vi "Set Shooter 2 RPM.vi"(8 "Open Loop":bool, 9 "Increment":bool, 10 "Decrement":bool, 11 "Shooter Enabled":bool) -> ()   [LabVIEW 2012]
uses:
  System Set Points and States.vi
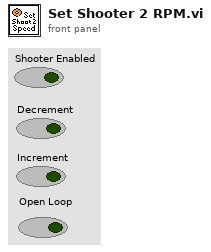
[diagram p1: front panel]
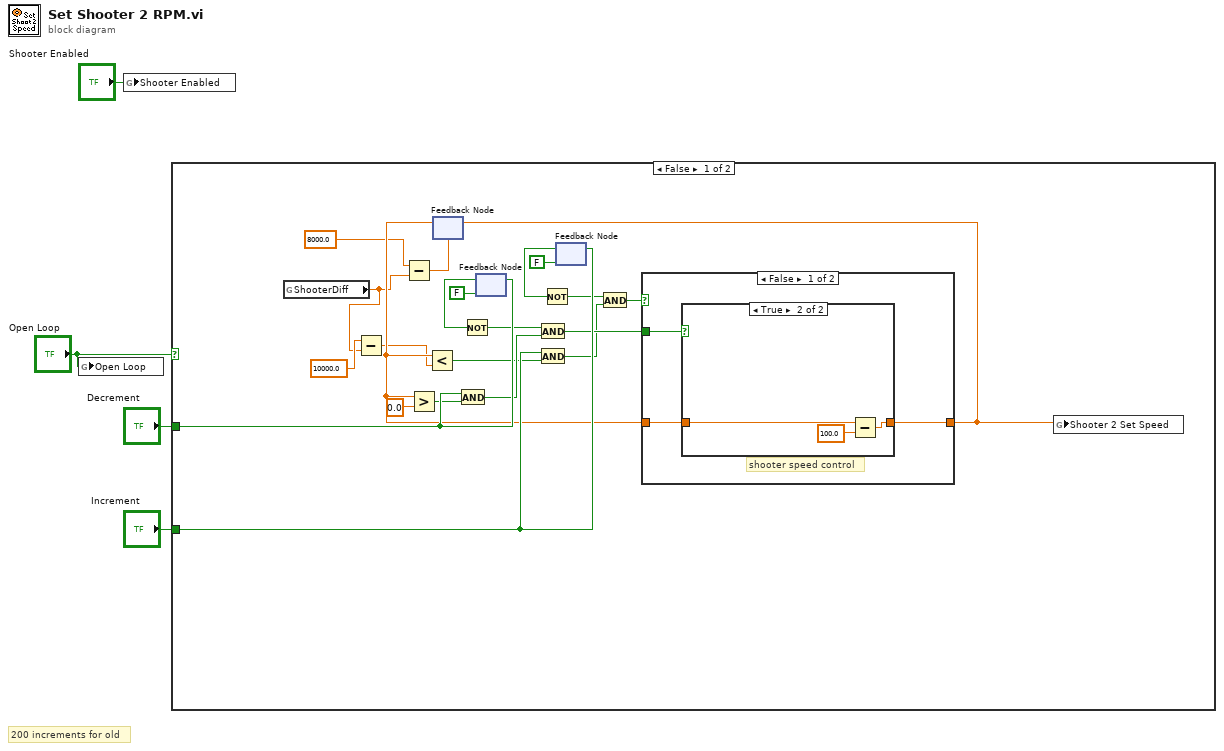
[diagram p0: block diagram]
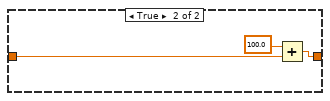
[diagram p3: hidden frame]
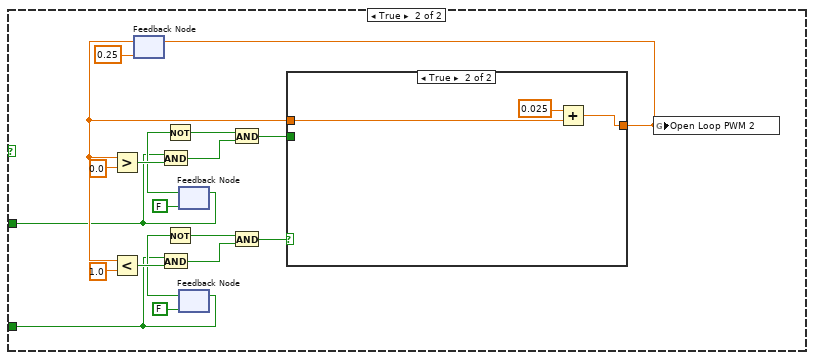
[diagram p4: hidden frame]
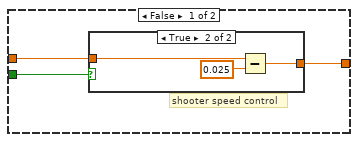
[diagram p5: hidden frame]
diagram:
  # "200 increments for old"
  n1 = global write "System Set Points and States.vi" "Open Loop"("Open Loop") -> ()
  n2 = global write "System Set Points and States.vi" "Shooter Enabled"("Shooter Enabled") -> ()
  n3 = case shown="False" "Open Loop" {
    tunnel: "Decrement" -> [w26 w39]
    tunnel: "Increment" -> [w25 w38]
    frame False {
      n4 = global read "System Set Points and States.vi" "ShooterDiff"() -> (w7:dbl)
      n5 = Subtract(x=10000.0 ("y"), y=w7) -> (x-y=w5:dbl)
      n6 = Subtract(x=8000.0, y=w7) -> (x-y=w6:dbl)
      n7 = feedback #1(w6) -> (w12:dbl)
      n8 = Greater?(x=w12, y=0.0) -> (0:w10:bool)
      n9 = Less?(x=w12, y=w5) -> (x < y?=w13:bool)
      n10 = And(x=w26, y=w10) -> (x .and. y?=w17:bool)
      n11 = feedback #2(FALSE) -> (w21:bool)
      n12 = Not(x=w21) -> (.not. x?=w22:bool)
      n13 = feedback-in #2(w26) -> ()
      n14 = And(x=w22, y=w17) -> (x .and. y?=w18:bool)
      n15 = And(x=w25, y=w13) -> (x .and. y?=w14:bool)
      n16 = feedback #3(FALSE) -> (w19:bool)
      n17 = Not(x=w19) -> (.not. x?=w20:bool)
      n18 = feedback-in #3(w25) -> ()
      n19 = And(x=w20, y=w14) -> (x .and. y?=w15:bool)
      n20 = case shown="False" w15 {
        tunnel: w18 -> [w29 _]
        tunnel: w12 -> [w28 w36]
        tunnel: [w27 w34] -> w24
        frame False {
          # "shooter speed control"
          n21 = case shown="True" w29 {
            tunnel: w28 -> [w30 w33]
            tunnel: [w30 w31] -> w27
            frame False {
            }
            frame True {
              n22 = Subtract(x=w33, y=100.0) -> (x-y=w31:dbl)
            }
          }
        }
        frame True {
          n23 = Add(x=100.0, y=w36) -> (x+y=w34:dbl)
        }
      }
      n24 = feedback-in #1(w24) -> ()
      n25 = global write "System Set Points and States.vi" "Shooter 2 Set Speed"(w24) -> ()
    }
    frame True {
      n26 = feedback #4(0.25) -> (w42:dbl)
      n27 = Greater?(x=w42, y=0.0) -> (0:w55:bool)
      n28 = Less?(x=w42, y=1.0) -> (x < y?=w53:bool)
      n29 = And(x=w39, y=w55) -> (x .and. y?=w48:bool)
      n30 = And(x=w38, y=w53) -> (x .and. y?=w50:bool)
      n31 = feedback #5(FALSE) -> (w45:bool)
      n32 = Not(x=w45) -> (.not. x?=w44:bool)
      n33 = feedback-in #5(w39) -> ()
      n34 = feedback #6(FALSE) -> (w47:bool)
      n35 = Not(x=w47) -> (.not. x?=w46:bool)
      n36 = feedback-in #6(w38) -> ()
      n37 = And(x=w44, y=w48) -> (x .and. y?=w41:bool)
      n38 = And(x=w46, y=w50) -> (x .and. y?=w40:bool)
      n39 = case shown="True" w40 {
        tunnel: w41 -> [w58 _]
        tunnel: w42 -> [w57 w65]
        tunnel: [w56 w63] -> w37
        frame False {
          # "shooter speed control"
          n40 = case shown="True" w58 {
            tunnel: w57 -> [w59 w62]
            tunnel: [w59 w60] -> w56
            frame False {
            }
            frame True {
              n41 = Subtract(x=w62, y=0.025) -> (x-y=w60:dbl)
            }
          }
        }
        frame True {
          n42 = Add(x=0.025, y=w65) -> (x+y=w63:dbl)
        }
      }
      n43 = feedback-in #4(w37) -> ()
      n44 = global write "System Set Points and States.vi" "Open Loop PWM 2"(w37) -> ()
    }
  }
